vi "Get Waveform Tasks.vi"(0 "Custom Device ref in":T2 format="%.0x", 3 "error in":errorcluster, 4 "UI Refs in":T1) -> (5 "UI Refs out":T1, 7 "Custom Device ref out":T2 format="%.0x", 10 "error out":errorcluster)   [LabVIEW 2017, in "Waveform-Processing-Custom-Device System Explorer.lvlib"]
uses:
  Waveform-Processing-Custom-Device System Explorer.lvlib
  <vilib>/NI Veristand/Custom Device API/Custom Device Item Ref.ctl
  Types/UI Refs Ctl.ctl
  NationalInstruments.VeriStand.SystemStorage
  <vilib>/NI VeriStand/Custom Device Tools/Custom Device Utility Library/Custom Device Utility Library.lvlib
  <vilib>/NI Veristand/Custom Device API/Custom Device API.lvlib
  Shared/Waveform-Processing-Custom-Device Shared.lvlib
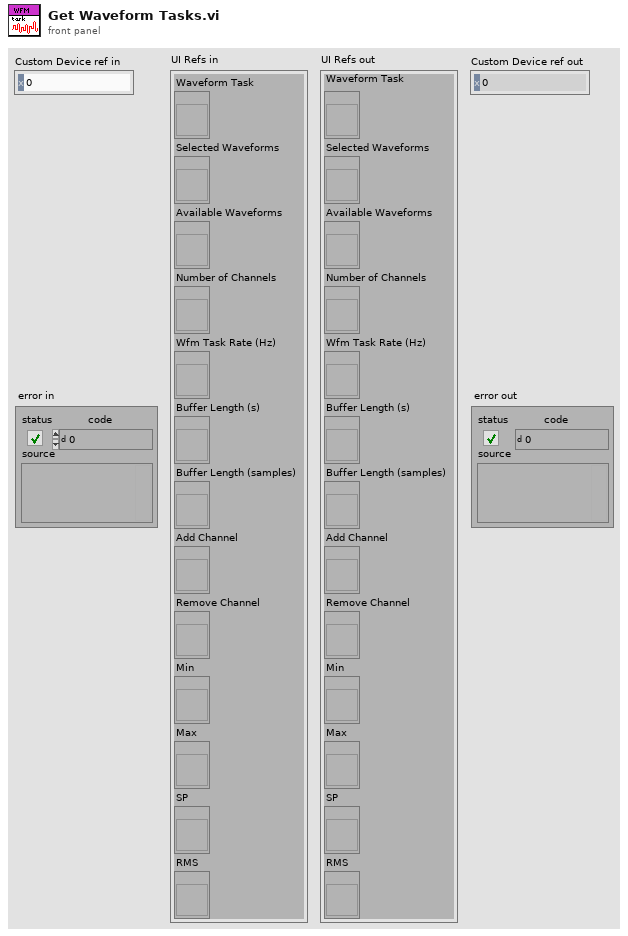
[diagram p1: front panel]
types:
  T1 = typedef "Waveform-Processing-Custom-Device Shared.lvlib/UI Refs Ctl.ctl" = cluster{"Waveform Task":refnum<vi>, "Selected Waveforms":refnum<vi>, "Available Waveforms":refnum<vi>, "Number of Channels":refnum<vi>, "Wfm Task Rate (Hz)":refnum<vi>, "Buffer Length (s)":refnum<vi>, "Buffer Length (samples)":refnum<vi>, "Add Channel":refnum<vi>, "Remove Channel":refnum<vi>, "Min":refnum<vi>, "Max":refnum<vi>, "SP":refnum<vi>, "RMS":refnum<vi>}
  T2 = typedef "Custom Device API.lvlib/Custom Device Item Ref.ctl" = u64
  T3 = typedef "Custom Device API.lvlib/Custom Device Pointer.ctl" = refnum<k24>
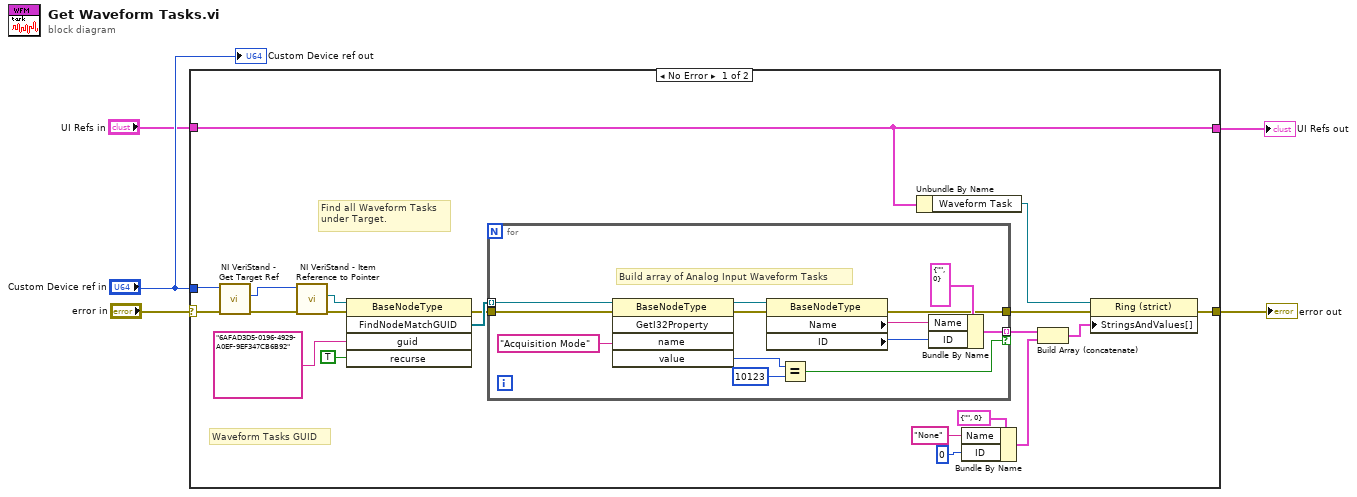
[diagram p0: block diagram]
diagram:
  n1 = case shown="No Error" "error in" {
    selector: "error in" -> [w16 w40]
    tunnel: [w8 w40] -> w4
    tunnel: "Custom Device ref in" -> [w15 _]
    tunnel: "UI Refs in" -> [w10 w39]
    tunnel: [w10 w39] -> w1
    frame No Error {
      # "Waveform Tasks GUID"
      # "Find all Waveform Tasks\nunder Target."
      n2 = call <vilib>:"NI VeriStand - Get Target Ref.vi"("error in"=w16, "Item Ref in"=w15) -> ("error out"=w14:errorcluster, "Target Ref"=w13:T2)  [unwired: 6 in, 2 out]
      n3 = call <vilib>:"NI VeriStand - Item Reference to Pointer.vi"("error in (no error)"=w14, "Item Ref in"=w13) -> ("error out"=w12:errorcluster, "Node Pointer"=w11:T3)  [unwired: 6 in, 2 out]
      n4 = invoke class="BaseNodeType" method="FindNodeMatchGUID"(reference=w11, error in=w12, "guid"="6AFAD3D5-0196-4929-A0EF-9EF347CB6B92", "recurse"=TRUE) -> (error out=w22:errorcluster, "FindNodeMatchGUID"=w23:refnum<k24>[])  [unwired: 1 in, 3 out]
      n5 = for {
        tunnel: w23 -> [w38] mode=indexing
        tunnel: w22 -> [w33]
        tunnel: [w28] -> w18 mode=indexing if=w27
        tunnel: [w26] -> w7
        # "Build array of Analog Input Waveform Tasks"
        n6 = invoke class="BaseNodeType" method="GetI32Property"(reference=w38, error in=w33, "name"="Acquisition Mode") -> (reference out=w36:refnum<k24>, error out=w34:errorcluster, "value"=w30:i32)  [unwired: 2 in, 2 out]
        n7 = property class="BaseNodeType"(reference=w36, error in=w34) -> (error out=w26:errorcluster, "Name"=w35:string, "ID"=w31:u64)  [unwired: 1 out]
        n8 = Equal?(x=w30, y=10123) -> (x = y?=w27:bool)
        n9 = Bundle By Name(cluster=cluster{"Name":string, "ID":u64} {"Name"="", "ID"=0} ("Waveform"), "Name"=w35, "ID"=w31) -> (w28:cluster{"Name":string, "ID":u64})
      }
      n10 = Unbundle By Name(w10) -> ("Waveform Task"=w9:refnum<vi>)
      n11 = Bundle By Name(cluster=cluster{"Name":string, "ID":u64} {"Name"="", "ID"=0} ("Waveform"), "Name"="None", "ID"=u64 0) -> (w17:cluster{"Name":string, "ID":u64})
      n12 = Build Array (concatenate)(w18, w17) -> (w6:cluster{"Name":string, "ID":u64}[])
      n13 = property class="Ring (strict)"(reference=w9, error in=w7, "StringsAndValues[]"=w6) -> (error out=w8:errorcluster)  [unwired: 1 out]
    }
    frame Error {
    }
  }
  "error out" <- w4
  "UI Refs out" <- w1
  "Custom Device ref out" <- "Custom Device ref in"
